vi "Delete.vi"(8 "error in (no error)":errorcluster, 11 "ARN in":refnum<class "ARN.lvclass">) -> (0 "error out":errorcluster)   [LabVIEW 2015, in "NI_AWS_Core.lvlib" / "ARN.lvclass"]
uses:
  ARN.lvclass
  HTTP Request/Name Value Pair.ctl
  HTTP Request/Request Options.ctl
  HTTP Request/Region handling.ctl
  HTTP Request/URL formatting.ctl
  ARN.lvclass/ARN.ctl
  Read ARN.vi
  HTTP Request/HTTP Request.lvclass
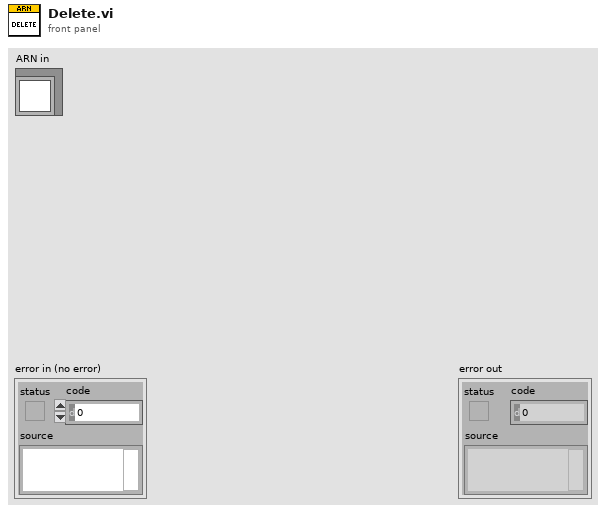
[diagram p1: front panel]
types:
  T1 = typedef "NI_AWS_Core.lvlib/HTTP Request.lvclass/Request Options.ctl" = cluster{"request headers":T2[], "request parameters":T2[], "request body":string, "region handling":T3, "URL formatting":T4}
  T2 = typedef "NI_AWS_Core.lvlib/HTTP Request.lvclass/Name Value Pair.ctl" = cluster{"name":string, "value":string}
  T3 = typedef "NI_AWS_Core.lvlib/HTTP Request.lvclass/Region handling.ctl" = enum16{"use region everywhere", "use region (authentication only)", "use region (URL only)", "ignore region everwhere"}
  T4 = typedef "NI_AWS_Core.lvlib/HTTP Request.lvclass/URL formatting.ctl" = enum16{"region-", "region."}
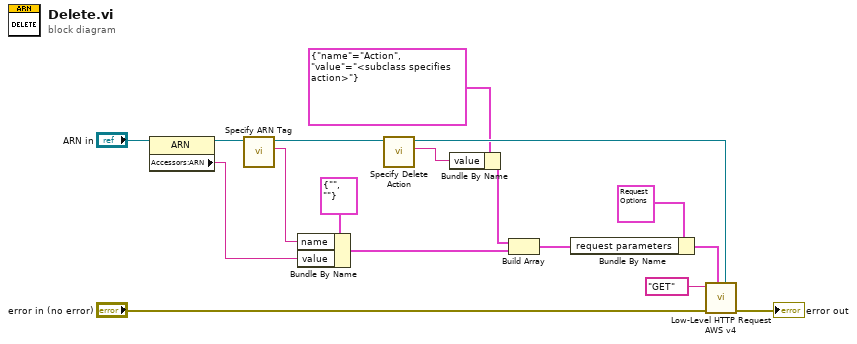
[diagram p0: block diagram]
diagram:
  n1 = property class="ARN"(reference="ARN in") -> (reference out=w9:refnum<class "ARN.lvclass">, "Accessors:ARN"=w13:string)  [unwired: 1 in, 1 out]
  n2 = call-dynamic "Specify ARN Tag.vi"("ARN in"=w9) -> ("ARN Tag"=w8:string, "ARN out"=w7:refnum<class "ARN.lvclass">)  [unwired: 9 in]
  n3 = Bundle By Name(cluster=T2 {"name"="", "value"=""} ("element"), "name"=w8, "value"=w13) -> (w15:T2)
  n4 = call-dynamic "Specify Delete Action.vi"("ARN in"=w7) -> ("Delete action"=w5:string, "ARN out"=w6:refnum<class "ARN.lvclass">)  [unwired: 9 in]
  n5 = Bundle By Name(cluster=T2 {"name"="Action", "value"="<subclass specifies action>"} ("Name Value Pair"), "value"=w5) -> (w3:T2)
  n6 = Build Array(w3, w15) -> (w14:T2[])
  n7 = Bundle By Name(cluster=T1 {"request headers"=[], "request parameters"=[], "request body"="", "region handling"=enum."use region everywhere", "URL formatting"=enum."region."} ("Request Options"), "request parameters"=w14) -> (w1:T1)
  n8 = call "Low-Level HTTP Request AWS v4.vi"("AWS Core"=w6, "Request Options"=w1, "error in (no error)"="error in (no error)", "HTTP-Verb"="GET") -> ("error out"=→"error out":errorcluster)  [unwired: 5 in, 2 out]
